vi "get desired keys.vi"(8 "error in":errorcluster, 11 "DAQmx Watchdog configuration in":refnum<class "DAQmx Watchdog configuration.lvclass">) -> (0 "error out":errorcluster, 2 "desired keys":string[](array[string]), 3 "DAQmx Watchdog configuration out":refnum<class "DAQmx Watchdog configuration.lvclass">)   [LabVIEW 2014, in "DAQmx Watchdog configuration.lvclass"]
uses:
  DAQmx Watchdog configuration.lvclass
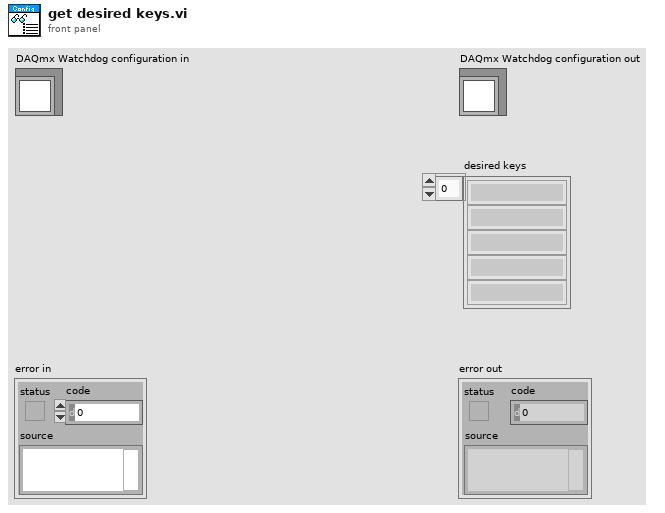
[diagram p1: front panel]
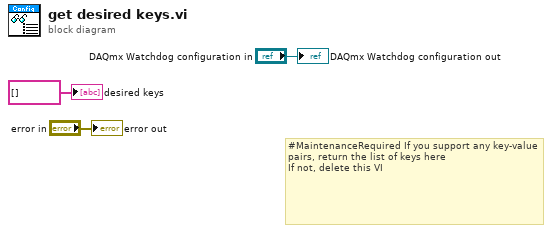
[diagram p0: block diagram]
diagram:
  # "#MaintenanceRequired If you support any key-value pairs, return the list of keys here\nIf not, delete this VI"
  "error out" <- "error in"
  "DAQmx Watchdog configuration out" <- "DAQmx Watchdog configuration in"
  "desired keys" <- string[] [] ("desired keys")
